vi "VisualizationTemplate.vi"() -> ()   [LabVIEW 2018]
doc: "This VI listens for any measurement data associated with the provided PluginName and displays it to the user for analysis. The display is only suitable for data coming from the RoomAlert Plugin."
uses:
  VisualizeBase/VisualizeBase_class/SubVIs/VisualizationOptions.ctl
  <vilib>/Utility/miscctls.llb/LVRectTypeDef.ctl
  VisualizeBase/VisualizeBase_class/Requests/VisUserEventType.ctl
  <vilib>/event_ctls.llb/usereventprio.ctl
  Sensor/SensorShared/clSensorData.ctl
  <extravilib>/ChannelInstances/Tag-bool/Read With Abort.vi
  <extravilib>/ChannelInstances/Tag-bool/Write With Abort.vi
  <extravilib>/ChannelInstances/Tag-bool/Instantiate.vi
  <extravilib>/ChannelInstances/Tag-bool/EndpointRead.vi
  <vilib>/Utility/error.llb/Error Cluster From Error Code.vi
  <extravilib>/ChannelInstances/Tag-bool/Endpoint.vi
  <vilib>/ErrorRing/Error Ring.xnode
  <userlib>/NIST/NISTErrorLib/NISTErrorLib.lvlib
  VisualizeBase/VisualizeBase_class/VisualizeBase.lvclass
  Sensor/SensorShared/SensorShared.lvlib
  Sensor/SensorModule/SensorModule.lvlib
  <extravilib>/ChannelInstances/Tag-bool.lvlib
  TestClass/Test.lvclass
  StatusAndLog/VisualizeStatus.lvclass
  Sensor/SensorPlugins/SensorPlugins.lvlib
panel:
  in  "btnPause":bool=TRUE
  out "VisualizationProperties":T1={"PauseAtStartup"=TRUE, "LogData"=FALSE, "LaunchInSubPanel"=TRUE, "FPMonitor"=0, "FPWindowBounds"={"Left"=0, "Top"=0, "Right"=0, "Bottom"=0}, "MonitorBounds"={"Left"=0, "Top"=0, "Right"=0, "Bottom"=0}}
  in  "INIFilePath":path
  in  "ModuleID":i32
  in  "Log Data":bool=TRUE
  in  "btnStop":bool
  in  "btnClearTest":bool
  in  "btnStopModule":bool
  out "ErrorArray":errorcluster[](array[cluster])
  out "String Results-Status":string="Sensor.RoomAlert1"
  in  "PluginName":string="Sensor.RoomAlert1"
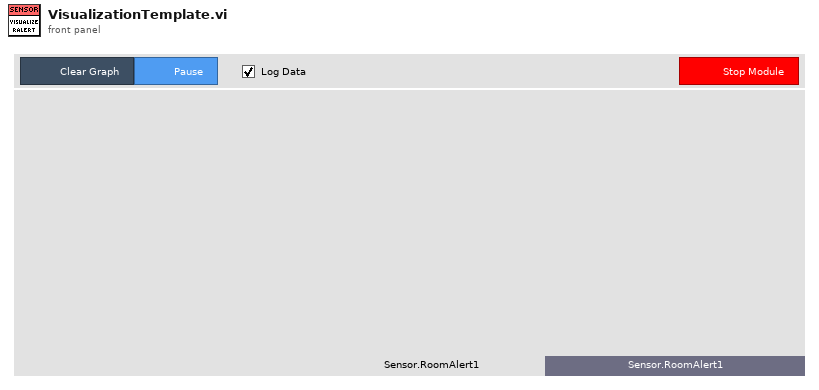
[diagram p1: front panel]
types:
  T1 = typedef "Visualization.lvlib/VisualizeBase.lvclass/VisualizationOptions.ctl" = cluster{"PauseAtStartup":bool, "LogData":bool, "LaunchInSubPanel":bool, "FPMonitor":u16, "FPWindowBounds":T2, "MonitorBounds":cluster{"Left":i16, "Top":i16, "Right":i16, "Bottom":i16}}
  T2 = typedef "LVRectTypeDef.ctl" = cluster{"Left":i16, "Top":i16, "Right":i16, "Bottom":i16}
  T3 = typedef "Visualization.lvlib/VisualizeBase.lvclass/VisRequestEvents.ctl" = cluster{"StopRequest":refnum<user-event>, "ResetRequest":refnum<user-event>, "FP Pop In or Out":refnum<user-event>}
  T4 = typedef "SensorShared.lvlib/clBroadcastEvents.ctl" = cluster{"DidInit":refnum<user-event>, "StatusUpdate":refnum<user-event>, "ErrorReport":refnum<user-event>, "DidStop":refnum<user-event>, "PathToINI":refnum<user-event>, "SensorReport":refnum<user-event>, "SensorConfig":refnum<user-event>}
  T5 = typedef "Visualization.lvlib/VisualizeBase.lvclass/VisFrmWrkBroadcastEvents.ctl" = cluster{"StatusUpdate":refnum<user-event>, "DidStop":refnum<user-event>, "NewModuleLoaded":refnum<user-event>, "StopVisualization":refnum<user-event>}
  T6 = enum16{"open", "open or create", "create or replace", "create", "open (read-only)"}
  T7 = typedef "SensorShared.lvlib/clSensorData.ctl" = cluster{"SensorType":string, "SensorData":variant, "TimeStamp":timestamp}
  T8 = typedef "Visualization.lvlib/VisualizeBase.lvclass/VisUserEventType.ctl" = cluster{"BusIndex":i8, "Data":variant}
  T9 = typedef "usereventprio.ctl" = enum32{"high priority", "normal priority"}
  T10 = typedef "Tag-bool.lvlib/))Channel.ctl" = refnum<queue>
  T11 = typedef "sizeaction.ctl" = enum32{"Minimized", "Maximized", "Resized"}
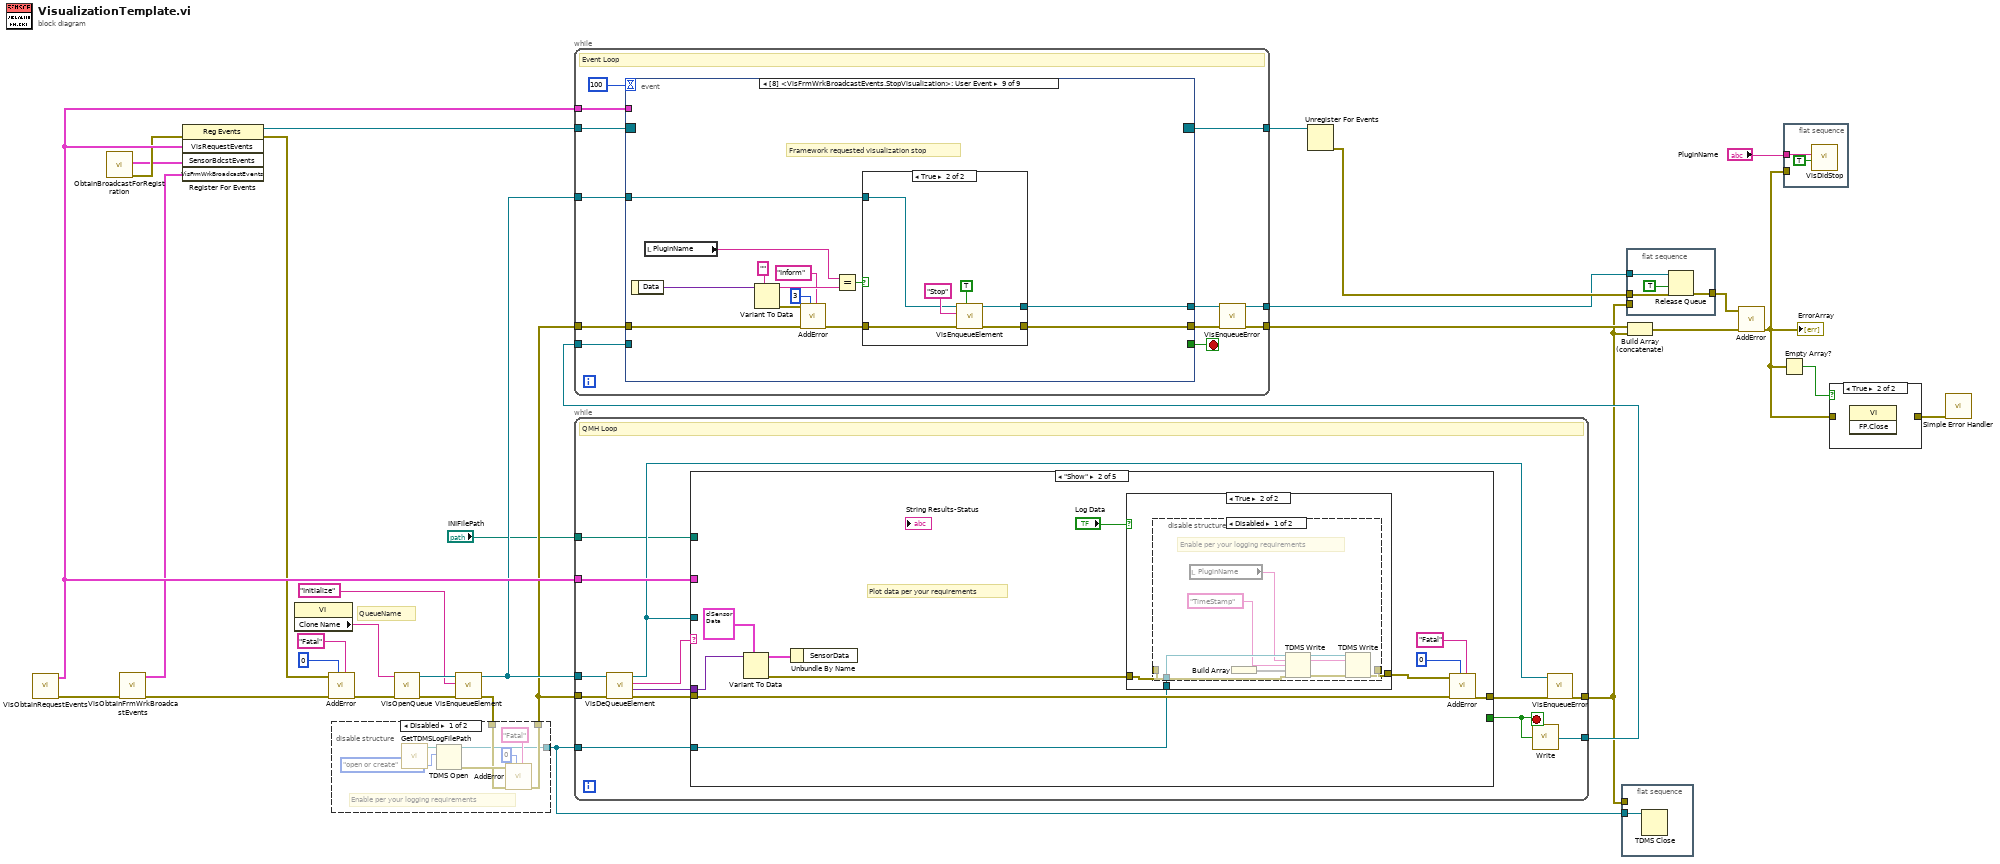
[diagram p0: block diagram]
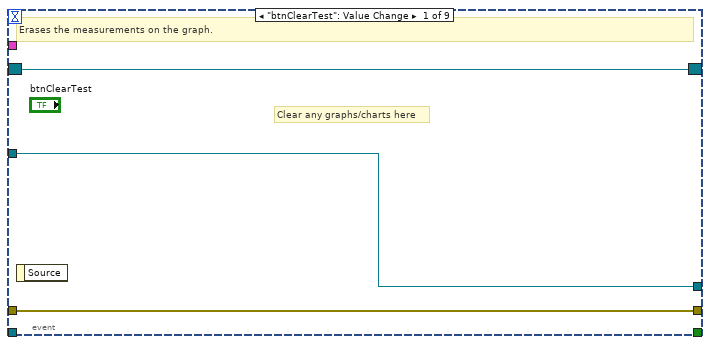
[diagram p3: hidden frame]
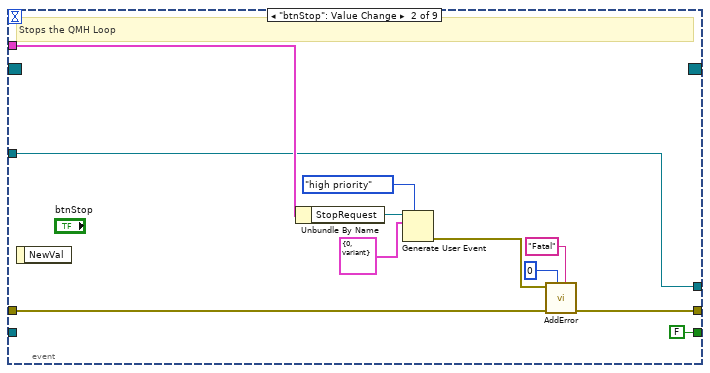
[diagram p4: hidden frame]
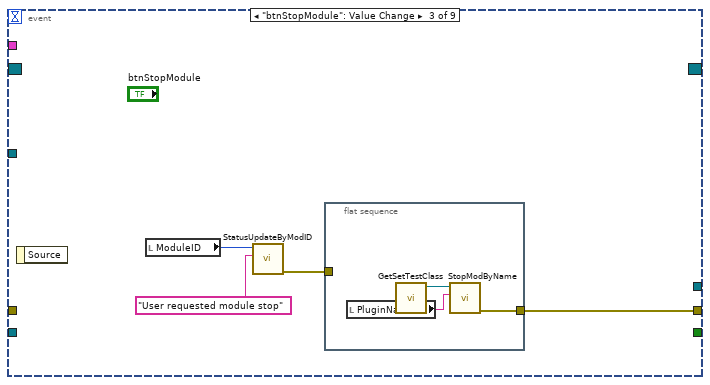
[diagram p5: hidden frame]
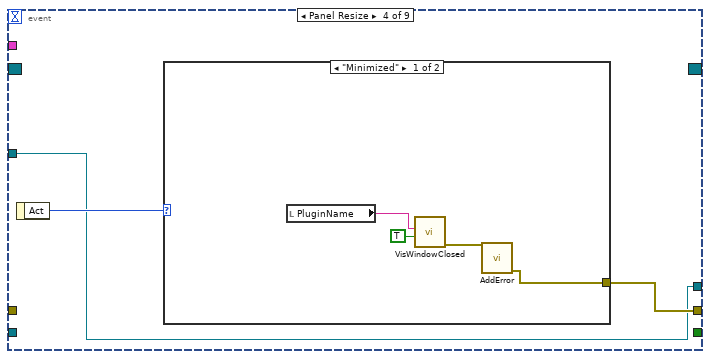
[diagram p6: hidden frame]
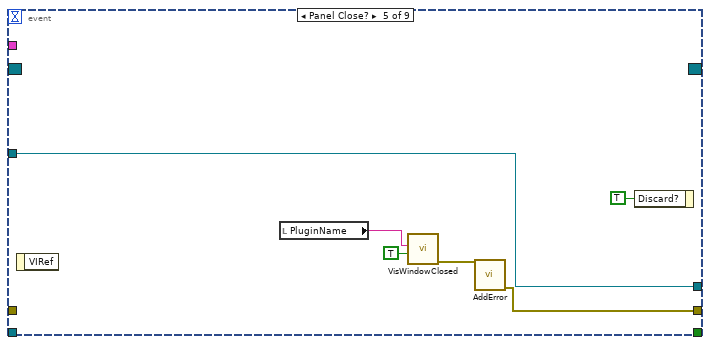
[diagram p8: hidden frame]
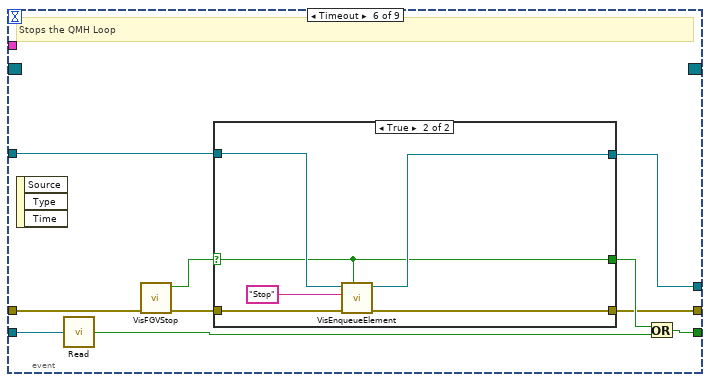
[diagram p9: hidden frame]
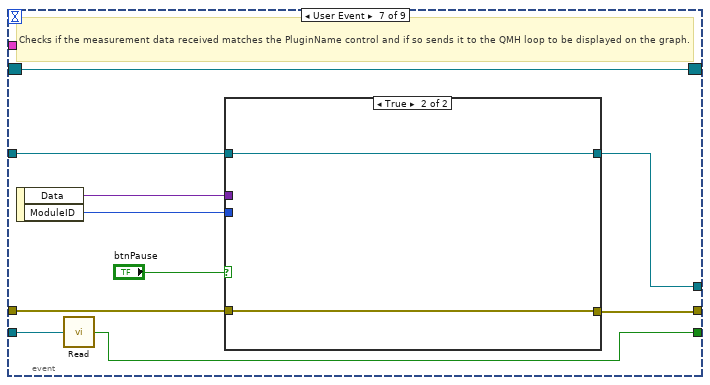
[diagram p11: hidden frame]
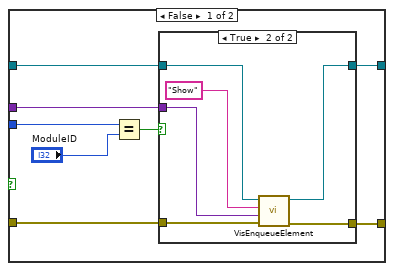
[diagram p12: hidden frame]
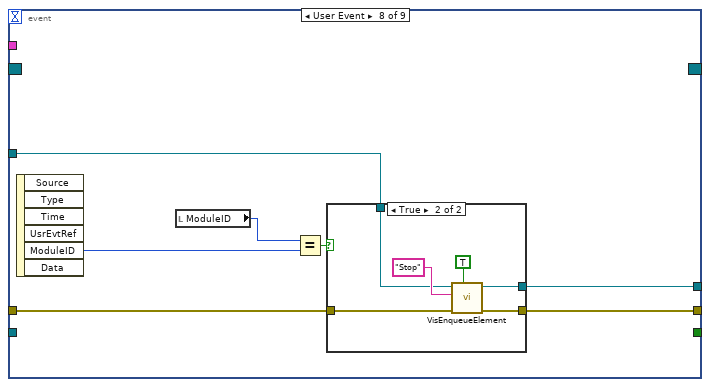
[diagram p14: hidden frame]
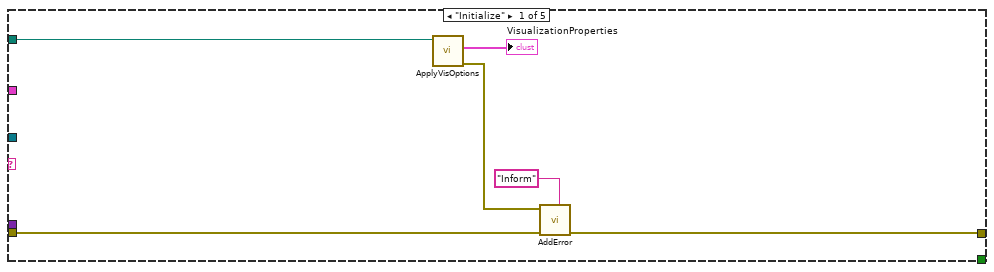
[diagram p17: hidden frame]
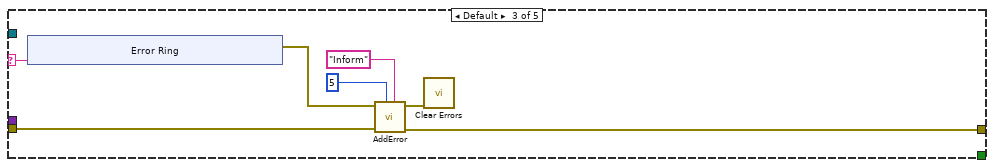
[diagram p20: hidden frame]
diagram:
  # "QueueName"
  n1 = call "VisObtainRequestEvents.vi"() -> ("Error"=w3:errorcluster[], "VisRequestEvents"=w25:T3)  [unwired: 10 in]
  n2 = call "ObtainBroadcastForRegistration.vi"() -> ("error out"=w20:errorcluster, "SensorBdcstEvents"=w12:T4)  [unwired: 10 in]
  n3 = call "VisObtainFrmWrkBroadcastEvents.vi"("Error"=w3) -> ("Error"=w2:errorcluster[], "VisFrmWrkBroadcastEvents"=w1:T5)  [unwired: 9 in]
  n4 = register-events(error in=w20, w25, w12, w1) -> (reference out=w32:refnum<event-registration>, error out=w23:errorcluster)  [unwired: 1 in]
  n5 = property class="VI"() -> ("Clone Name"=w10:string)  [unwired: 2 in, 2 out]
  n6 = call <userlib>:"AddError.vi"("Severity"="Fatal", "Priority"=u8 0, "ErrorArray In"=w2, "error in (no error)"=w23) -> ("ErrorArray Out"=w19:errorcluster[])  [unwired: 6 in, 1 out]
  n7 = call "VisOpenQueue.vi"("Error Array In"=w19, "QueueName"=w10) -> ("Error Array Out"=w17:errorcluster[], "queue out"=w18:refnum<queue>)  [unwired: 8 in]
  n8 = call "VisEnqueueElement.vi"("Error Array In"=w17, "Message"="Initialize", "queue in"=w18) -> ("Error Array Out"=w9:errorcluster[], "queue out"=w15:refnum<queue>)  [unwired: 7 in]
  n9 = disable-structure shown="Disabled" {
    disable-tunnel: w9 -> [w36 w41]
    disable-tunnel: [w35 w41] -> w8
    disable-tunnel: [w33 _] -> w7
    frame Disabled {
      # "Enable per your logging requirements"
      n10 = call "GetTDMSLogFilePath.vi"() -> ("TDMS Log File Path"=w40:path)  [unwired: 11 in]
      n11 = TDMS Open(10:T6."open or create" ("operation (0:open)"), 11:w40) -> (0:w37:errorcluster, 3:w33:refnum<k34>)  [unwired: 5 in]
      n12 = call <userlib>:"AddError.vi"("Severity"="Fatal", "Priority"=u8 0, "ErrorArray In"=w36, "error in (no error)"=w37) -> ("ErrorArray Out"=w35:errorcluster[])  [unwired: 6 in, 1 out]
    }
    frame Enabled {
    }
  }
  n13 = while {
    tunnel: w8 -> [w48]
    tunnel: [w51] -> w6
    tunnel: w15 -> [w47]
    tunnel: w25 -> [w53]
    tunnel: [w44] -> w11
    tunnel: w7 -> [w43]
    tunnel: "INIFilePath" -> [w42]
    stop <- w54 stop-if-true
    # "QMH Loop"
    n14 = call "VisDeQueueElement.vi"("Error Array In"=w48, "Queue In"=w47) -> ("Error Array Out"=w46:errorcluster[], "Data"=w49:variant, "Message"=w50:string, "Queue Out"=w45:refnum<queue>)  [unwired: 6 in]
    n15 = case shown="\"Show\"" w50 {
      selector: w50 -> [_ _ w91 _ _]
      tunnel: w49 -> [_ w67 _ w110 _]
      tunnel: w46 -> [w57 w70 w89 _ w139]
      tunnel: [w58 w71 w88 w100 w138] -> w52
      tunnel: [_ _ _ w106 TRUE] -> w54
      tunnel: w53 -> [_ _ _ w105 _]
      tunnel: w45 -> [_ _ _ w104 _]
      tunnel: w43 -> [_ w61 _ _ _]
      tunnel: w42 -> [w56 _ _ _ w140]
      frame "Initialize" {
        n16 = call "ApplyVisOptions.vi"("INIFilePath"=w56) -> ("error out"=w60:errorcluster, "VisualizationProperties"=→"VisualizationProperties":T1)  [unwired: 9 in]
        n17 = call <userlib>:"AddError.vi"("Severity"="Inform", "ErrorArray In"=w57, "error in (no error)"=w60) -> ("ErrorArray Out"=w58:errorcluster[])  [unwired: 7 in, 1 out]
      }
      frame "Show" {
        # "Plot data per your requirements"
        n18 = Variant To Data(type=T7 {"SensorType"="", "SensorData"=variant, "TimeStamp"=timestamp(0 s since 1904-01-01)} ("clSensorData"), Variant=w67) -> (data=w65:T7, error out=w66:errorcluster)  [unwired: 1 in]
        n19 = Unbundle By Name(w65) -> ()  [unwired: 1 out]
        n20 = case shown="True" "Log Data" {
          tunnel: w66 -> [w72 w74]
          tunnel: [w72 w75] -> w63
          tunnel: w61 -> [_ w73]
          frame False {
          }
          frame True {
            n21 = disable-structure shown="Disabled" {
              disable-tunnel: [w84 _] -> w75
              disable-tunnel: w74 -> [w83 _]
              disable-tunnel: w73 -> [w81 _]
              frame Disabled {
                # "Enable per your logging requirements"
                n22 = local read "PluginName"() -> (w79:string)
                n23 = Build Array() -> (w76:void[])  [unwired: 1 in]
                n24 = TDMS Write(0:w81, 5:w79, 7:"TimeStamp" ("PluginName"), 9:w76, 11:w83) -> (4:w80:refnum<k34>, 6:w78:string, 15:w82:errorcluster)  [unwired: 1 in, 1 out]
                n25 = TDMS Write(0:w80, 5:w78, 11:w82) -> (15:w84:errorcluster)  [unwired: 3 in, 3 out]
              }
              frame Enabled {
              }
            }
          }
        }
        n26 = call <userlib>:"AddError.vi"("Severity"="Fatal" ("String"), "Priority"=u8 0, "ErrorArray In"=w70, "error in (no error)"=w63) -> ("ErrorArray Out"=w71:errorcluster[])  [unwired: 6 in, 1 out]
      }
      frame Default {
        n27 = xnode "Error Ring"("parameter 0"=w91) -> ("error out"=w90:errorcluster)
        n28 = call <userlib>:"AddError.vi"("Severity"="Inform" ("String"), "Priority"=u8 5, "ErrorArray In"=w89, "error in (no error)"=w90) -> ("ErrorArray Out"=w88:errorcluster[], "error out"=w87:errorcluster)  [unwired: 6 in]
        n29 = call <vilib>:"Clear Errors.vi"("error in (no error)"=w87) -> ()  [unwired: 5 in, 2 out]
      }
      frame "Error" {
        n30 = Variant To Data(type=errorcluster[] [], Variant=w110) -> (data=w108:errorcluster[], error out=w99:errorcluster)  [unwired: 1 in]
        n31 = call <userlib>:"ParseErrors.vi"("ErrorArray"=w108) -> ("ErrorArray"=w107:errorcluster[])  [unwired: 8 in, 2 out]
        n32 = for {
          tunnel: w107 -> [w121] mode=indexing
          tunnel: [w115] -> w101 mode=concatenating
          tunnel: [w113] -> w106
          tunnel: w105 -> [w112]
          tunnel: w104 -> [w111]
          stop <- w113 stop-if-true
          n33 = call <userlib>:"GeneralHandler.vi"("error in (no error)"=w121) -> ("Severity"=w114:string, "Stop"=w118:bool, "Abort"=w119:bool, "Continue"=w120:bool)  [unwired: 6 in, 1 out]
          n34 = Build Array(w120, w119, w118) -> (w117:bool[])
          n35 = Boolean Array To Number(Boolean array=w117) -> (number=w116:u32)
          n36 = case shown="1" w116 {
            tunnel: [_ _ w126 w135] -> w115
            tunnel: w114 -> [_ _ _ w128]
            tunnel: [_ _ _ w130] -> w113
            tunnel: w112 -> [_ _ _ w129]
            tunnel: w111 -> [_ _ w122 _]
            frame 0, Default {
              # "No Dialog"
            }
            frame 1 {
              # "Continue"
            }
            frame 2 {
              # "Abort, Flush Queue"
              n37 = Flush Queue(queue=w122) -> (error out=w125:errorcluster)  [unwired: 1 in, 2 out]
              n38 = call <userlib>:"AddError.vi"("Severity"="Critical" ("String"), "Priority"=u8 1, "error in (no error)"=w125) -> ("ErrorArray Out"=w126:errorcluster[])  [unwired: 7 in, 1 out]
            }
            frame 4 {
              # "Stop"
              n39 = Unbundle By Name(w129) -> ("StopRequest"=w136:refnum<user-event>)
              n40 = Equal?(x=w128, y="Fatal" ("x")) -> (x = y?=w130:bool)
              n41 = Generate User Event(priority (normal)=usereventprio."high priority", user event=w136, event data cluster=T8 {"BusIndex"=0, "Data"=variant} ("event data")) -> (error out=w134:errorcluster)  [unwired: 1 in, 1 out]
              n42 = call <userlib>:"AddError.vi"("error in (no error)"=w134) -> ("ErrorArray Out"=w135:errorcluster[], "error out"=w131:errorcluster)  [unwired: 9 in]
              n43 = call <vilib>:"Clear Errors.vi"("error in (no error)"=w131) -> ()  [unwired: 5 in, 2 out]
            }
          }
        }
        n44 = call <userlib>:"AddError.vi"("Severity"="Critical", "Priority"=u8 2, "ErrorArray In"=w101, "error in (no error)"=w99) -> ("ErrorArray Out"=w100:errorcluster[])  [unwired: 6 in, 1 out]
      }
      frame "Stop" {
        n45 = local read "VisualizationProperties"() -> (w137:T1)
        n46 = call "WriteVisOptionsToINIFile.vi"("Visualization Options"=w137, "INIFilePath"=w140) -> ("error out"=w141:errorcluster)  [unwired: 8 in, 1 out]
        n47 = call <userlib>:"AddError.vi"("Severity"="Inform", "ErrorArray In"=w139, "error in (no error)"=w141) -> ("ErrorArray Out"=w138:errorcluster[])  [unwired: 7 in, 1 out]
      }
    }
    n48 = call <extravilib>:"Write.vi"("element"=w54) -> ("channel"=w44:T10)  [unwired: 1 out]
    n49 = call "VisEnqueueError.vi"("Error Array In"=w52, "Queue in"=w45) -> ("Error Array Out"=w51:errorcluster[])  [unwired: 8 in, 1 out]
  }
  n50 = while {
    tunnel: w32 -> [w155]
    tunnel: [w149] -> w30
    tunnel: [w153] -> w31
    tunnel: w25 -> [w152]
    tunnel: w8 -> [w151]
    tunnel: w15 -> [w150]
    tunnel: [w146] -> w14
    tunnel: w11 -> [w144]
    stop <- w154 stop-if-true
    # "Event Loop"
    n51 = event shown="[8] <VisFrmWrkBroadcastEvents.StopVisualization>: User Event" {
      selector: w155 -> [w157 _ _ _ _ _ w214 _ _]
      dyn-events: [w157 _ _ _ _ _ w214 _ _] -> w153
      timeout: 100 -> [_ _ _ _ _ _ _ _ _]
      tunnel: [_ FALSE ("Priority? (F)") _ _ _ w190 w211 _ _] -> w154
      tunnel: [w158 w162 w173 w178 w185 w192 w216 w240 w258] -> w148
      tunnel: w152 -> [_ w161 _ _ _ _ _ _ _]
      tunnel: w151 -> [w158 w169 _ _ _ w195 w217 w239 w256]
      tunnel: w150 -> [w156 w159 _ w177 w184 w194 w218 w242 w260]
      tunnel: [w156 w159 _ w177 w184 w193 w215 w241 w254] -> w147
      tunnel: w144 -> [_ _ _ _ _ w199 w212 _ _]
      event "btnClearTest": Value Change {
        # "Clear any graphs/charts here"
        # "Erases the measurements on the graph."
        n52 = event-data() -> ()  [unwired: 1 in, 1 out]
      }
      event "btnStop": Value Change {
        # "Stops the QMH Loop"
        n53 = event-data() -> ()  [unwired: 1 in, 1 out]
        n54 = Unbundle By Name(w161) -> ("StopRequest"=w167:refnum<user-event>)
        n55 = Generate User Event(priority (normal)=usereventprio."high priority", user event=w167, event data cluster=T8 {"BusIndex"=0, "Data"=variant} ("event data")) -> (error out=w168:errorcluster)  [unwired: 1 in, 1 out]
        n56 = call <userlib>:"AddError.vi"("Severity"="Fatal" ("String"), "Priority"=u8 0, "ErrorArray In"=w169, "error in (no error)"=w168) -> ("ErrorArray Out"=w162:errorcluster[])  [unwired: 6 in, 1 out]
      }
      event "btnStopModule": Value Change {
        n57 = event-data() -> ()  [unwired: 1 in, 1 out]
        n58 = local read "ModuleID"() -> (w172:i32)
        n59 = call "StatusUpdateByModID.vi"("Status"="User requested module stop", "Accessors:Module ID"=w172) -> ("error out"=w171:errorcluster)  [unwired: 9 in]
        n60 = flat-sequence {
          tunnel: [w175] -> w173
          tunnel: w171 -> [_]
          frame #0 {
            n61 = local read "PluginName"() -> (w174:string)
            n62 = call "GetSetTestClass.vi"() -> ("Test.lvclass"=w176:refnum<class "Test.lvclass">)  [unwired: 11 in]
            n63 = call "StopModByName.vi"("Module Name"=w174, "Test.lvclass"=w176) -> ("ErrorArray Out"=w175:errorcluster[])  [unwired: 4 in, 5 out]
          }
        }
      }
      event Panel Resize {
        n64 = event-data() -> ("Act"=w179:T11)  [unwired: 1 in]
        n65 = case shown="\"Minimized\"" w179 {
          tunnel: [w180 _] -> w178
          frame "Minimized" {
            n66 = local read "PluginName"() -> (w182:string)
            n67 = call "VisWindowClosed.vi"("Window Closed?"=TRUE ("Window Minimized or Clozed?"), "Module Name"=w182) -> ("error out"=w183:errorcluster)  [unwired: 9 in]
            n68 = call <userlib>:"AddError.vi"("error in (no error)"=w183) -> ("ErrorArray Out"=w180:errorcluster[])  [unwired: 9 in, 1 out]
          }
          frame "Maximized", Default {
          }
        }
      }
      event Panel Close? {
        n69 = event-data() -> ()  [unwired: 1 in, 1 out]
        n70 = local read "PluginName"() -> (w186:string)
        n71 = call "VisWindowClosed.vi"("Window Closed?"=TRUE ("Window Minimized or Clozed?"), "Module Name"=w186) -> ("error out"=w187:errorcluster)  [unwired: 9 in]
        n72 = call <userlib>:"AddError.vi"("error in (no error)"=w187) -> ("ErrorArray Out"=w185:errorcluster[])  [unwired: 9 in, 1 out]
        n73 = event-data("Discard?"=TRUE) -> ()  [unwired: 1 in, 1 out]
      }
      event Timeout {
        # "Stops the QMH Loop"
        n74 = event-data() -> ()  [unwired: 1 in, 3 out]
        n75 = call <extravilib>:"Read.vi"("channel"=w199) -> ("element"=w191:bool)  [unwired: 1 in, 1 out]
        n76 = call "VisFGVStop.vi"("Error In"=w195) -> ("Error Out"=w197:errorcluster[], "Value"=w198:bool)  [unwired: 9 in]
        n77 = case shown="True" w198 {
          selector: w198 -> [w200 w203]
          tunnel: [w202 w206] -> w192
          tunnel: w197 -> [w202 w207]
          tunnel: w194 -> [w201 w205]
          tunnel: [w201 w204] -> w193
          tunnel: [w200 w203] -> w196
          frame False {
          }
          frame True {
            n78 = call "VisEnqueueElement.vi"("Priority? (F)"=w203, "Error Array In"=w207, "Message"="Stop", "queue in"=w205) -> ("Error Array Out"=w206:errorcluster[], "queue out"=w204:refnum<queue>)  [unwired: 6 in]
          }
        }
        n79 = Or(x=w196, y=w191) -> (x .or. y?=w190:bool)
      }
      event User Event {
        # "Checks if the measurement data received matches the PluginName control and if so sends it to the QMH loop to be displayed on the graph."
        n80 = event-data() -> ("Data"=w213:variant, "ModuleID"=w210:i32)  [unwired: 1 in]
        n81 = call <extravilib>:"Read.vi"("channel"=w212) -> ("element"=w211:bool)  [unwired: 1 in, 1 out]
        n82 = case shown="True" "btnPause" {
          tunnel: w218 -> [w226 w236]
          tunnel: w217 -> [w225 w235]
          tunnel: [w224 w235] -> w216
          tunnel: [w223 w236] -> w215
          tunnel: w213 -> [w222 _]
          tunnel: w210 -> [w219 _]
          frame False {
            n83 = Equal?(x=w219, y="ModuleID") -> (x = y?=w221:bool)
            n84 = case shown="True" w221 {
              tunnel: [w227 w233] -> w224
              tunnel: w226 -> [w228 w232]
              tunnel: w225 -> [w227 w234]
              tunnel: [w228 w230] -> w223
              tunnel: w222 -> [_ w231]
              frame False {
              }
              frame True {
                n85 = call "VisEnqueueElement.vi"("Error Array In"=w234, "Data"=w231, "Message"="Show", "queue in"=w232) -> ("Error Array Out"=w233:errorcluster[], "queue out"=w230:refnum<queue>)  [unwired: 6 in]
              }
            }
          }
          frame True {
          }
        }
      }
      event User Event {
        n86 = event-data() -> ("ModuleID"=w238:i32)  [unwired: 1 in, 5 out]
        n87 = local read "ModuleID"() -> (w237:i32)
        n88 = Equal?(x=w237, y=w238) -> (x = y?=w243:bool)
        n89 = case shown="True" w243 {
          tunnel: [w244 w249] -> w240
          tunnel: [w245 w248] -> w241
          tunnel: w242 -> [w245 w247]
          tunnel: w239 -> [w244 w246]
          frame False {
          }
          frame True {
            n90 = call "VisEnqueueElement.vi"("Priority? (F)"=TRUE, "Error Array In"=w246, "Message"="Stop", "queue in"=w247) -> ("Error Array Out"=w249:errorcluster[], "queue out"=w248:refnum<queue>)  [unwired: 6 in]
          }
        }
      }
      event User Event {
        # "Framework requested visualization stop"
        n91 = event-data() -> ("Data"=w264:variant)  [unwired: 1 in]
        n92 = local read "PluginName"() -> (w261:string)
        n93 = Variant To Data(type="" ("Message"), Variant=w264) -> (data=w262:string, error out=w257:errorcluster)  [unwired: 1 in]
        n94 = call <userlib>:"AddError.vi"("Severity"="Inform", "Priority"=u8 3, "ErrorArray In"=w256, "error in (no error)"=w257) -> ("ErrorArray Out"=w255:errorcluster[])  [unwired: 6 in, 1 out]
        n95 = Equal?(x=w261, y=w262) -> (x = y?=w259:bool)
        n96 = case shown="True" w259 {
          tunnel: w260 -> [w266 w270]
          tunnel: [w265 w269] -> w258
          tunnel: w255 -> [w265 w268]
          tunnel: [w266 w267] -> w254
          frame False {
          }
          frame True {
            n97 = call "VisEnqueueElement.vi"("Priority? (F)"=TRUE, "Error Array In"=w268, "Message"="Stop", "queue in"=w270) -> ("Error Array Out"=w269:errorcluster[], "queue out"=w267:refnum<queue>)  [unwired: 6 in]
          }
        }
      }
    }
    n98 = call "VisEnqueueError.vi"("Error Array In"=w148, "Queue in"=w147) -> ("Error Array Out"=w149:errorcluster[], "Queue out"=w146:refnum<queue>)  [unwired: 8 in]
  }
  n99 = Unregister For Events(event registration refnum=w31) -> (error out=w29:errorcluster)  [unwired: 1 in]
  n100 = flat-sequence {
    tunnel: w7 -> [w273]
    tunnel: w6 -> [_]
    frame #0 {
      n101 = TDMS Close(11:w273) -> ()  [unwired: 1 in, 2 out]
    }
  }
  n102 = flat-sequence {
    tunnel: w29 -> [w277]
    tunnel: [w276] -> w27
    tunnel: w14 -> [w275]
    tunnel: w6 -> [_]
    frame #0 {
      n103 = Release Queue(queue=w275, force destroy? (F)=TRUE, error in (no error)=w277) -> (error out=w276:errorcluster)  [unwired: 2 out]
    }
  }
  n104 = Build Array (concatenate)(w30, w6) -> (w28:errorcluster[])
  n105 = call <userlib>:"AddError.vi"("ErrorArray In"=w28, "error in (no error)"=w27) -> ("ErrorArray Out"=w26:errorcluster[])  [unwired: 8 in, 1 out]
  "ErrorArray" <- w26
  n106 = Empty Array?(array=w26) -> (empty?=w24:bool)
  n107 = flat-sequence {
    tunnel: "PluginName" -> [w279]
    tunnel: w26 -> [_]
    frame #0 {
      n108 = call "VisDidStop.vi"("DidStop?"=TRUE, "Module Name"=w279) -> ()  [unwired: 9 in, 1 out]
    }
  }
  n109 = case shown="True" w24 {
    tunnel: [w280 _] -> w13
    tunnel: w26 -> [w281 _]
    frame False {
      n110 = Merge Errors(w281) -> (w280:errorcluster)
    }
    frame True {
      n111 = invoke class="VI" method="FP.Close"() -> ()  [unwired: 3 in, 3 out]
    }
  }
  n112 = call <vilib>:"Simple Error Handler.vi"("error in (no error)"=w13) -> ()  [unwired: 4 in, 5 out]
